vi "Shutdown.vi"   [LabVIEW 2019]
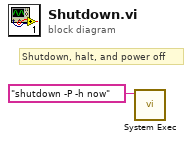
[diagram p0: block diagram]
diagram:
  # "Shutdown, halt, and power off"
  n1 = call <vilib>:"System Exec.vi"("command line"="shutdown -P -h now") -> ()  [unwired: 7 in, 4 out]
